vi "Computation.vi"(0 "offset":dbl, 5 "Operand 1":dbl, 9 "Operand 2":dbl) -> (4 "Result":dbl)   [LabVIEW 2021, in "Meas B.lvlib"]
uses:
  Meas B.lvlib
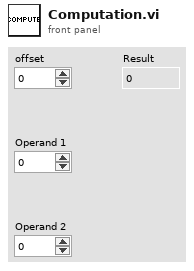
[diagram p1: front panel]
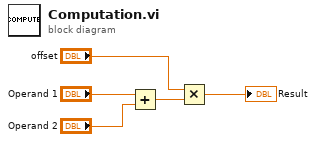
[diagram p0: block diagram]
diagram:
  n1 = Add(x="Operand 1", y="Operand 2") -> (x+y=w3:dbl)
  n2 = Multiply(x="offset", y=w3) -> (x*y=→"Result":dbl)
